vi "Interval Trigger 03.vi"(5 "First Call?: T/F":bool, 6 "Iteration#":i32, 8 "Loop mS":u32, 9 "Interval Sec":u32=5) -> (0 "Go":bool, 3 "Timestamp sec":u32, 4 "1st iteration#":i32)   [LabVIEW 2020]
panel:
  out "Iter/Interval":u32
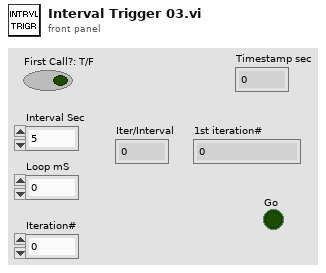
[diagram p1: front panel]
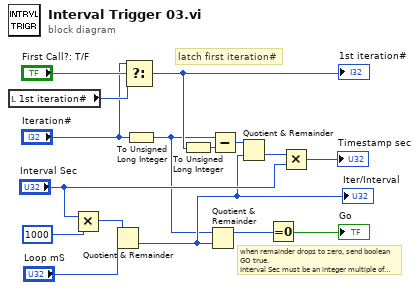
[diagram p0: block diagram]
diagram:
  # "when remainder drops to zero, send boolean GO true.\nInterval Sec must be an integer multiple of loop mS"
  # "latch first iteration#"
  n1 = local read "1st iteration#"() -> (w11:i32)
  n2 = Multiply(x="Interval Sec", y=u32 1000) -> (x*y=w15:u32)
  n3 = Quotient & Remainder(x=w15, y="Loop mS") -> (floor(x/y)=w5:u32)  [unwired: 1 out]
  "Iter/Interval" <- w5
  n4 = Select(t="Iteration#", s="First Call?: T/F", f=w11) -> (s? t:f=w13:i32)
  "1st iteration#" <- w13
  n5 = To Unsigned Long Integer(number="Iteration#") -> (unsigned 32bit integer=w2:u32)
  n6 = To Unsigned Long Integer(number=w13) -> (unsigned 32bit integer=w1:u32)
  n7 = Quotient & Remainder(x=w2, y=w5) -> (x-y*floor(x/y)=w8:u32)  [unwired: 1 out]
  n8 = Subtract(x=w2, y=w1) -> (x-y=w4:u32)
  n9 = Quotient & Remainder(x=w4, y=w5) -> (floor(x/y)=w3:u32)  [unwired: 1 out]
  n10 = Equal To 0?(x=w8) -> (x = 0?=→"Go":bool)
  n11 = Multiply(x=w3, y="Interval Sec") -> (x*y=→"Timestamp sec":u32)
